vi "混合信号图.vi"() -> ()   [LabVIEW 2010]
uses:
  <vilib>/Waveform/DWDTOps.llb/Digital Pattern Generator (Random).vi
  <vilib>/measure/NI_MABase.lvlib
panel:
  out "混合信号图":T1(graph)
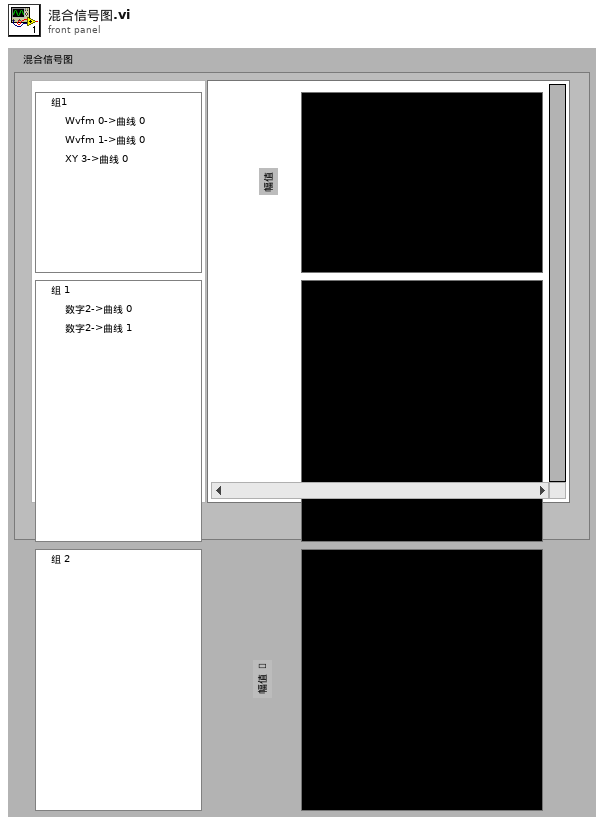
[diagram p1: front panel]
types:
  T1 = cluster{"signal out":waveform(dbl), dbl[], "digital waveform":digitalwaveform, cluster{dbl[], dbl[]}}
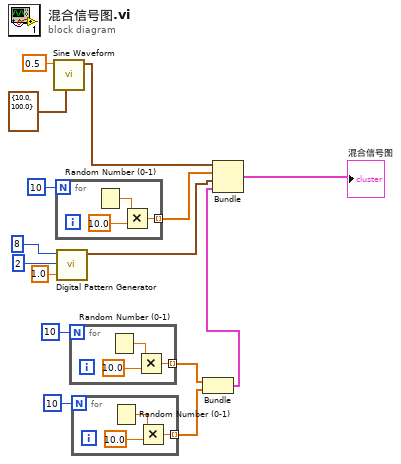
[diagram p0: block diagram]
diagram:
  n1 = call <vilib>:"Sine Waveform.vi"("sampling info"=cluster{"Fs":dbl, "#s":dbl} {"Fs"=10.0, "#s"=100.0}, "frequency"=0.5) -> ("signal out"=w13:waveform(dbl))  [unwired: 8 in, 1 out]
  n2 = for {
    N: 10 -> [_]
    tunnel: [w16] -> w11 mode=indexing
    n3 = Random Number (0-1)() -> (number: 0 to 1=w18:dbl)
    n4 = Multiply(x=w18, y=10.0) -> (x*y=w16:dbl)
  }
  n5 = call-poly <vilib>:"Digital Pattern Generator.vi"("sample rate"=1.0, "number of signals"=u32 2, "number of samples"=u32 8) -> ("digital waveform"=w7:digitalwaveform)  [unwired: 7 in, 1 out]
  n6 = for {
    N: 10 -> [_]
    tunnel: [w19] -> w3 mode=indexing
    n7 = Random Number (0-1)() -> (number: 0 to 1=w21:dbl)
    n8 = Multiply(x=w21, y=10.0) -> (x*y=w19:dbl)
  }
  n9 = for {
    N: 10 -> [_]
    tunnel: [w22] -> w2 mode=indexing
    n10 = Random Number (0-1)() -> (number: 0 to 1=w24:dbl)
    n11 = Multiply(x=w24, y=10.0) -> (x*y=w22:dbl)
  }
  n12 = Bundle(w3, w2) -> (w1:cluster{dbl[], dbl[]})  [unwired: 1 in]
  n13 = Bundle("signal out"=w13, w11, "digital waveform"=w7, w1) -> (→"混合信号图":T1)  [unwired: 1 in]
